vi "OPN csv .vi"(8 "error in (no error)":errorcluster, 11 "文件路径":path) -> (0 "error out":errorcluster, 3 "data":string[][](array[string]))   [LabVIEW 2019, in "Instrument.lvclass"]
uses:
  Instrument.lvclass
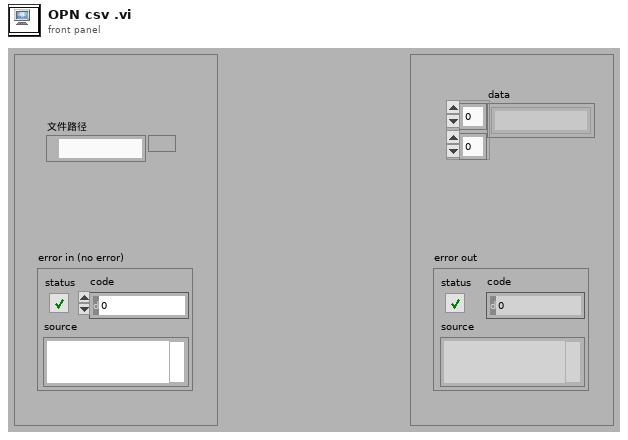
[diagram p1: front panel]
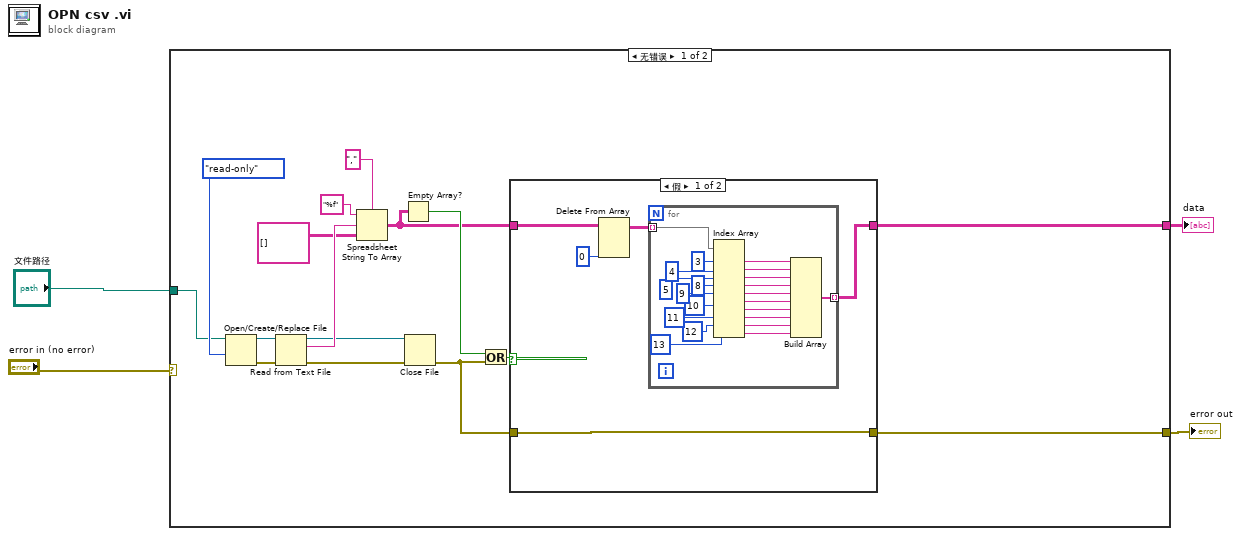
[diagram p0: block diagram]
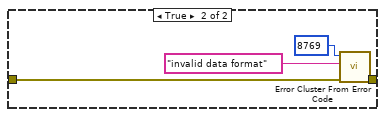
[diagram p2: hidden frame]
diagram:
  n1 = case shown="无错误" "error in (no error)" {
    selector: "error in (no error)" -> [_ w51]
    tunnel: [w20 w51] -> w4
    tunnel: [w19 _] -> w1
    tunnel: "文件路径" -> [w6 _]
    frame No Error {
      n2 = Open/Create/Replace File(file path (use dialog)=w6, access (0:read/write)=enum16{"read/write", "read-only", "write-only"}."read-only") -> (refnum out=w17:refnum<file>, error out=w16:errorcluster)  [unwired: 4 in, 1 out]
      n3 = Read from Text File(file (use dialog)=w17, error in=w16) -> (refnum out=w8:refnum<file>, text=w14:string, error out=w15:errorcluster)  [unwired: 2 in, 1 out]
      n4 = Spreadsheet String To Array(delimiter (Tab)=",", format string="%f", spreadsheet string=w14, array type (2D Dbl)=string[][] []) -> (array=w9:string[][])
      n5 = Empty Array?(array=w9) -> (empty?=w11:bool)
      n6 = Close File(refnum=w8, error in=w15) -> (error out=w10:errorcluster)  [unwired: 1 out]
      n7 = Or(x=w11, y=w10) -> (x .or. y?=w7:bool)
      n8 = case shown="假" w7 {
        tunnel: [w23 w49] -> w20
        tunnel: w10 -> [w23 w50]
        tunnel: w9 -> [w25 _]
        tunnel: [w21 _] -> w19
        frame False {
          n9 = Delete From Array(array=w25, index (row)=0 ("索引 (行)")) -> (array with subset deleted=w22:string[][])  [unwired: 2 in, 1 out]
          n10 = for {
            tunnel: w22 -> [w46] mode=indexing
            tunnel: [w35] -> w21 mode=indexing
            n11 = Index Array(array=w46, index #1=3 ("索引"), index #2=4 ("索引"), index #3=5 ("索引"), index #4=8 ("索引"), index #5=9 ("索引"), index #6=10 ("索引"), index #7=11 ("索引"), index #9=12 ("索引"), index #10=13 ("索引")) -> (element #1=w45:string, element #2=w44:string, element #3=w43:string, element #4=w42:string, element #5=w41:string, element #6=w40:string, element #7=w39:string, element #8=w38:string, element #9=w37:string, element #10=w36:string)  [unwired: 1 in]
            n12 = Build Array(w45, w44, w43, w42, w41, w40, w39, w38, w37, w36) -> (w35:string[])
          }
        }
        frame True {
          n13 = call <vilib>:"Error Cluster From Error Code.vi"("error in (no error)"=w50, "error message (\"\")"="invalid data format" ("error message (\"\")"), "error code (0)"=8769) -> ("error out"=w49:errorcluster)  [unwired: 6 in]
        }
      }
    }
    frame Error {
    }
  }
  "error out" <- w4
  "data" <- w1
